vi "Get Fiducials.vi"(6 "error in":errorcluster, 7 "Image Prefix":string, 8 "Fiducial Type":T1, 9 "CameraTool In":refnum<class "CameraTool Class.lvclass">) -> (0 "error out":errorcluster, 1 "Fiducial Image":T2, 2 "Fiducial Image Positions":refnum<class "Vec3d Class.lvclass">[](array[class]), 3 "CameraTool Out":refnum<class "CameraTool Class.lvclass">)   [LabVIEW 2011, in "CameraTool Class.lvclass"]
doc: "This VI looks for fiducials in input images. It returns the number of fiducials found in the input image and a list of up to 10 x,y pairs of fiducial locations in the image.\n\nImage Name can be given if multiple images are wanted to be collected. Otherwise, the image must be disposed of before calling again."
uses:
  CameraTool Class.lvclass
  Vec3d Class/Vec3d Class.lvclass
  Utils/Type Definitions/Physical Image.ctl
  <vilib>/vision/Image Controls.llb/IMAQ Image.ctl
  Config Manager Class/Type Definitions/Fiducial Type.ctl
  Config Manager Class/Type Definitions/Camera Enum.ctl
  gVision API/gVision/gVision.lvlib
  Config Manager Class/Config Manager Class.lvclass
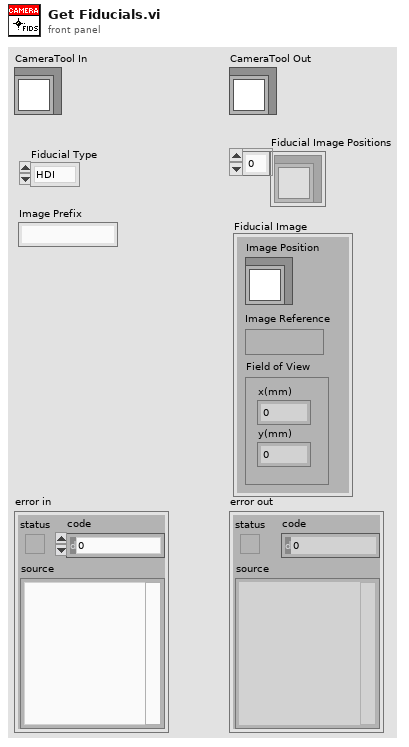
[diagram p1: front panel]
types:
  T1 = typedef "Fiducial Type.ctl" = enum16{"HDI", "BBM"}
  T2 = typedef "Physical Image.ctl" = cluster{"Image Position":refnum<class "Vec3d Class.lvclass">, "Image Reference":T3, "Field of View":cluster{"x(mm)":dbl, "y(mm)":dbl}}
  T3 = typedef "IMAQ Image.ctl" = refnum<image>
  T4 = typedef "Camera Enum.ctl" = enum16{"GANTRY HEAD", "NEEDLE CALIBRATION X", "NEEDLE CALIBRATION Y"}
  T5 = typedef "Fiducial Finder Parameters.ctl" = cluster{"shrinkFactor":sgl, "dilateSize":i32, "sizeMin":sgl, "sizeMax":sgl, "arMin":sgl, "arMax":sgl, "colorGroups":i32, "maxAttempts":i32}
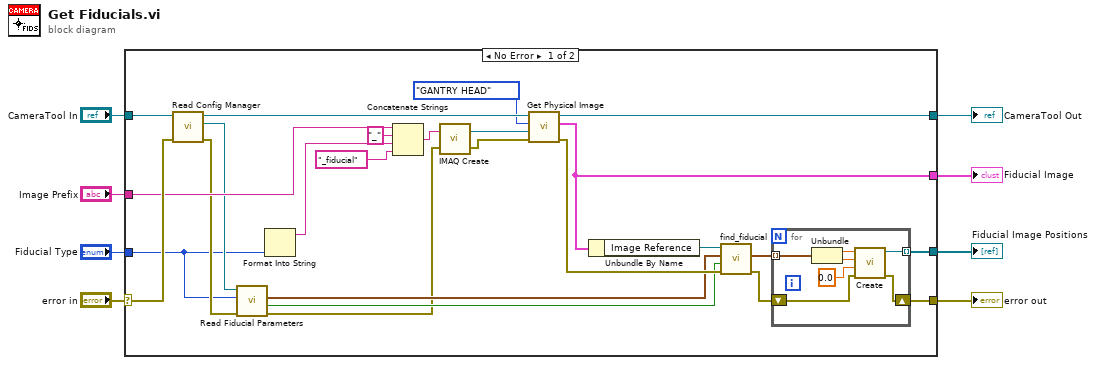
[diagram p0: block diagram]
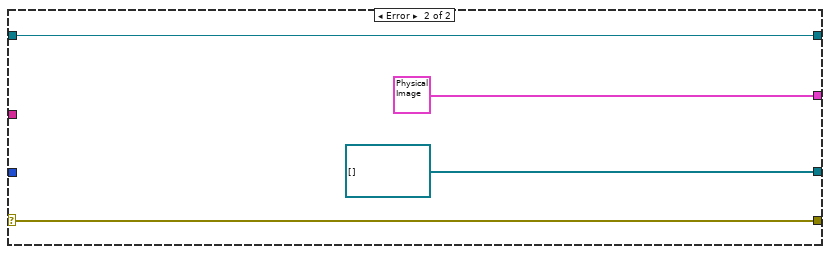
[diagram p2: hidden frame]
diagram:
  n1 = case shown="No Error" "error in" {
    selector: "error in" -> [w33 w44]
    tunnel: [w30 w44] -> w7
    tunnel: "CameraTool In" -> [w27 w43]
    tunnel: [w32 w43] -> w5
    tunnel: [w31 refnum<class "Vec3d Class.lvclass">[] []] -> w4
    tunnel: [w29 T2 {"Image Position"=refnum, "Image Reference"=refnum, "Field of View"={"x(mm)"=0.0, "y(mm)"=0.0}} ("Physical Image")] -> w3
    tunnel: "Image Prefix" -> [w28 _]
    tunnel: "Fiducial Type" -> [w15 _]
    frame No Error {
      n2 = call-dynamic "Read Config Manager.vi"("error in"=w33, "Gantry in"=w27) -> ("error out"=w16:errorcluster, "Config Manager"=w17:refnum<class "Config Manager Class.lvclass">, "Gantry out"=w26:refnum<class "CameraTool Class.lvclass">)  [unwired: 7 in]
      n3 = call "Read Fiducial Parameters.vi"("error in"=w16, "Fiducial Type"=w15, "Config Manager in"=w17) -> ("error out"=w11:errorcluster, "Interactive Mode"=w12:bool, "Fiducial Parameters"=w13:T5)  [unwired: 5 in, 1 out]
      n4 = Format Into String(w15) -> (resulting string=w14:string)  [unwired: 3 in, 1 out]
      n5 = Concatenate Strings(w28, "_" ("string"), w14, "_fiducial" ("string")) -> (w20:string)
      n6 = call "IMAQ Create"("Image Name"=w20, "error in (no error)"=w11) -> ("New Image"=w22:T3, "error out"=w10:errorcluster)  [unwired: 3 in]
      n7 = call-dynamic "Get Physical Image.vi"("error in"=w10, "Image In"=w22, "Camera Name"=Camera_Enum."GANTRY HEAD", "Gantry in"=w26) -> ("error out"=w24:errorcluster, "Physical Image"=w29:T2, "Gantry out"=w32:refnum<class "CameraTool Class.lvclass">)  [unwired: 5 in]
      n8 = Unbundle By Name(w29) -> ("Image Reference"=w21:T3)
      n9 = call "find_fiducial.vi"("error in"=w24, "interactive"=w12, "Fiducial Parameters"=w13, "Image"=w21) -> ("error out"=w25:errorcluster, "coords"=w23:cluster{"x":dbl, "y":dbl}[])  [unwired: 6 in]
      n10 = for {
        tunnel: [w40] -> w31 mode=indexing
        shift-right: [w38] -> w30
        shift-left: w25 -> [w39]
        tunnel: w23 -> [w36] mode=indexing
        n11 = Unbundle(w36) -> ("x"=w35:dbl, "y"=w34:dbl)
        n12 = call "Create.vi"("error in"=w39, "Z"=0.0, "Y"=w34, "X"=w35) -> ("error out"=w38:errorcluster, "Vec3d Class out"=w40:refnum<class "Vec3d Class.lvclass">)  [unwired: 6 in]
      }
    }
    frame Error {
    }
  }
  "error out" <- w7
  "CameraTool Out" <- w5
  "Fiducial Image Positions" <- w4
  "Fiducial Image" <- w3
